vi "AmmeterInit.vi"(8 "error in (no error)":errorcluster, 11 "VISA resource name":refnum<visa-resource-name>="GPIB1::22::INSTR") -> (0 "error out":errorcluster, 3 "VISA resource name out":refnum<visa-resource-name>)   [LabVIEW 2012]
uses:
  Agilent 34401.lvlib
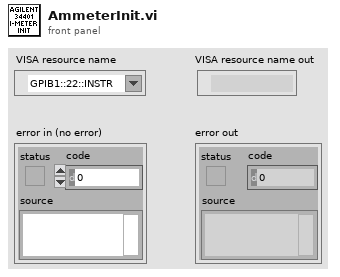
[diagram p1: front panel]
types:
  T1 = cluster{"Baud Rate":u32, "Parity":u16, "Data Bits":u16}
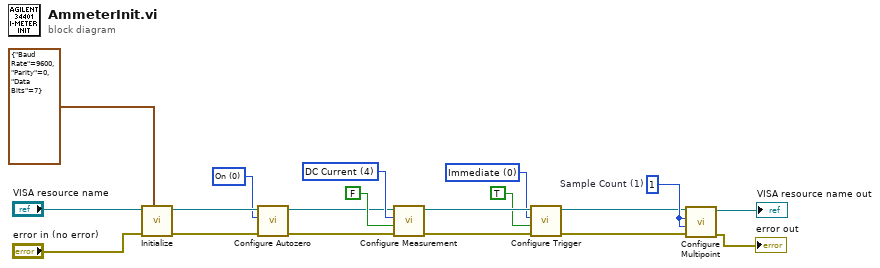
[diagram p0: block diagram]
diagram:
  w4 = u16 0 items=["On", "Off", "Once"] ("Autozero  (0: On)")
  w11 = 1  # Sample Count (1)
  w12 = u16 0 items=["Immediate", "Software (Bus)", "External", "Internal"] ("Trigger Source (0: Immediate)")
  w16 = u16 4 items=["DC Voltage", "AC Voltage", "2 - Wire Resistance", "4 - Wire Resistance", "DC Current", "AC Current", "Frequency", "Period", "Continuity", "Diode Checking", "VDC:VDC Ratio", "Temperature", "Capacitance"] ("Function (0: DC Voltage)")
  n1 = call "Initialize.vi"("Serial Configuration"=T1 {"Baud Rate"=9600, "Parity"=0, "Data Bits"=7}, "error in (no error)"="error in (no error)", "VISA resource name"="VISA resource name") -> ("error out"=w6:errorcluster, "VISA resource name out"=w8:refnum<visa-resource-name>)  [unwired: 7 in]
  n2 = call "Configure Autozero.vi"("error in (no error)"=w6, "Autozero  (0: On)"=w4, "VISA resource name"=w8) -> ("error out"=w5:errorcluster, "VISA resource name out"=w7:refnum<visa-resource-name>)  [unwired: 7 in]
  n3 = call "Configure Measurement.vi"("error in (no error)"=w5, "Enable Auto Range (T: Enable)"=FALSE, "Function (0: DC Voltage)"=w16, "VISA resource name"=w7) -> ("error out"=w13:errorcluster, "VISA resource name out"=w14:refnum<visa-resource-name>)  [unwired: 6 in]
  n4 = call "Configure Trigger.vi"("error in (no error)"=w13, "Enable Auto Delay (T: Enable)"=TRUE, "Trigger Source (0: Immediate)"=w12, "VISA resource name"=w14) -> ("error out"=w9:errorcluster, "VISA resource name out"=w10:refnum<visa-resource-name>)  [unwired: 6 in]
  n5 = call "Configure Multipoint.vi"("error in (no error)"=w9, "Sample Count (1)"=w11, "Trigger Count (1)"=w11, "VISA resource name"=w10) -> ("error out"=→"error out":errorcluster, "VISA resource name out"=→"VISA resource name out":refnum<visa-resource-name>)  [unwired: 6 in]
